vi "Test Multitone.vi"() -> ()   [LabVIEW 2019, in "Instrument.DAQ.lvclass"]
uses:
  Instrument.DAQ.lvclass
  <vilib>/measure/NI_MAPro.lvlib
  <vilib>/measure/NI_MABase.lvlib
panel:
  out "timer 0 (ms)":u32
  out "timer 3 (ms)":u32
  out "timer 2 (ms)":u32
  out "timer 1 (ms)":u32
  out "Waveform Graph":waveform(dbl)[](graph)
  out "resulting string":string
  in  "phase":dbl[](array[numeric])
  in  "frequency":dbl[](array[numeric])
  in  "amplitude":dbl[](array[numeric])
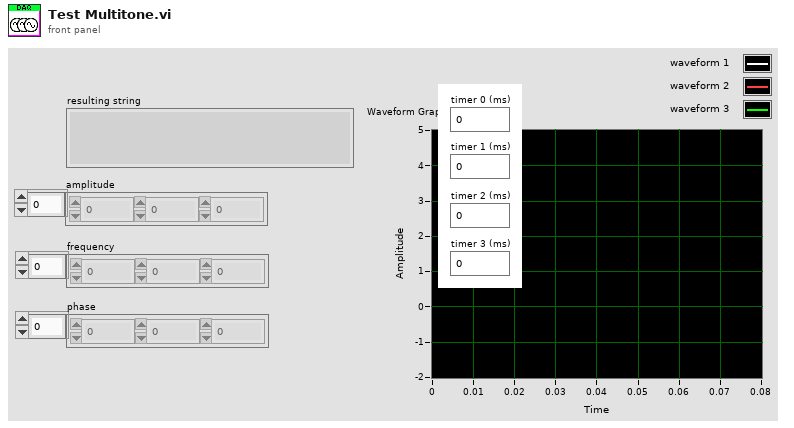
[diagram p1: front panel]
types:
  T1 = enum16{"Sine Wave", "Triangle Wave", "Square Wave", "Sawtooth Wave"}
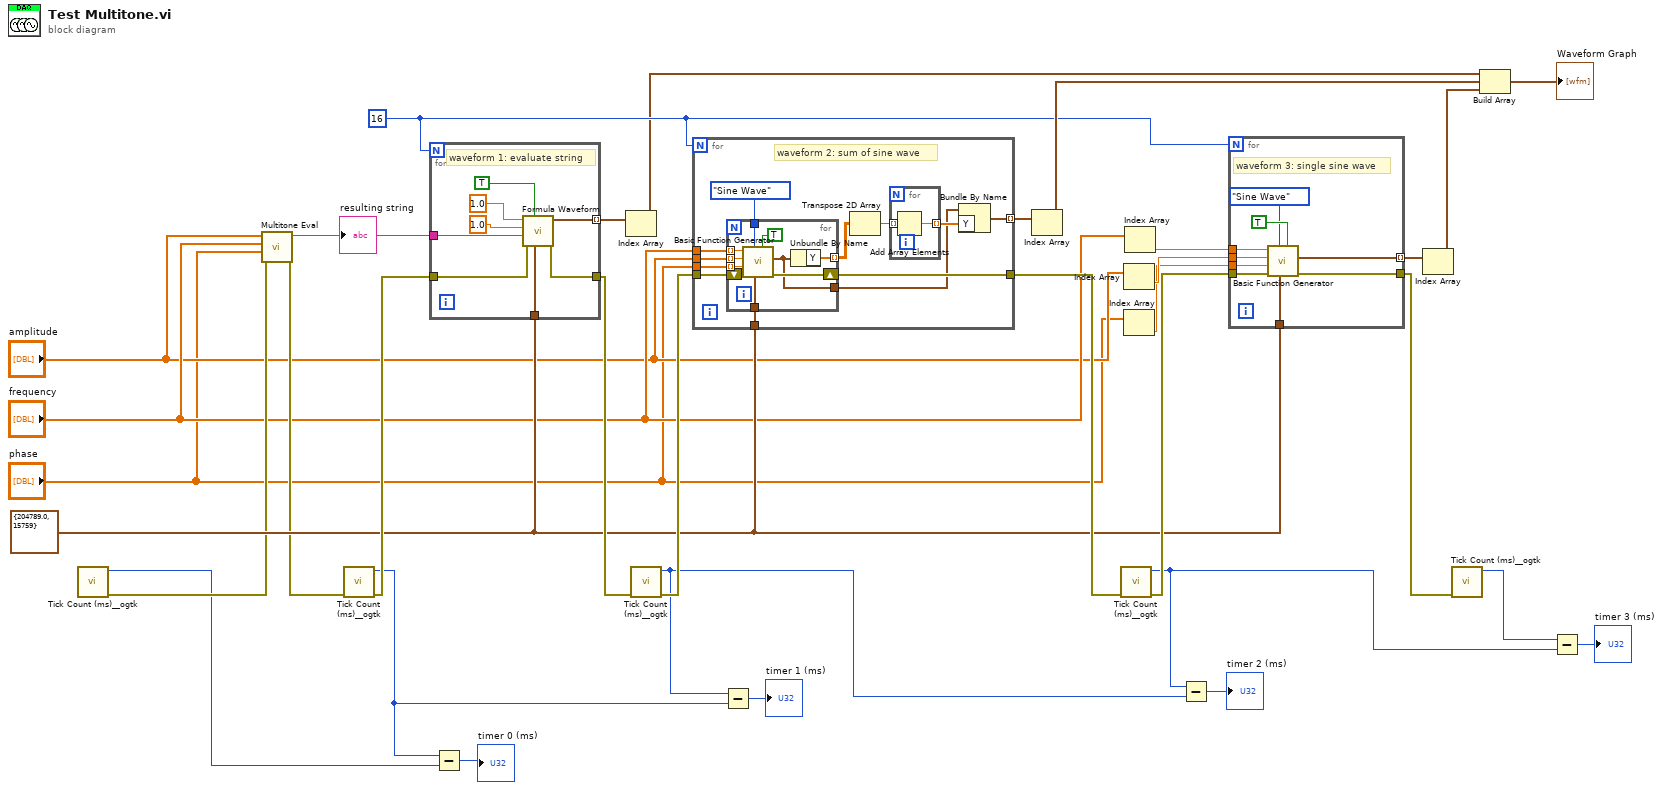
[diagram p0: block diagram]
diagram:
  w9 = 16
  w28 = cluster{"Fs":dbl, "#s":i32} {"Fs"=204789.0, "#s"=15759} ("sampling")
  n1 = call <userlib>:"Tick Count (ms)__ogtk.vi"() -> ("error out"=w26:errorcluster, "millisecond timer value"=w2:u32)  [unwired: 10 in]
  n2 = call "Multitone Eval.vi"("error in (no error)"=w26, "phase"="phase", "frequency"="frequency", "amplitude"="amplitude") -> ("error out"=w25:errorcluster, "String"=w24:string)  [unwired: 6 in]
  "resulting string" <- w24
  n3 = call <userlib>:"Tick Count (ms)__ogtk.vi"("error in (no error)"=w25) -> ("error out"=w33:errorcluster, "millisecond timer value"=w3:u32)  [unwired: 9 in]
  n4 = for {
    N: w9 -> [_]
    tunnel: w28 -> [w41]
    tunnel: w24 -> [w40]
    tunnel: w33 -> [w36]
    tunnel: [w35] -> w32
    tunnel: [w34] -> w23 mode=indexing
    # "waveform 1: evaluate string"
    n5 = call <vilib>:"Formula Waveform.vi"("sampling info"=w41, "reset signal"=TRUE, "error in (no error)"=w36, "formula"=w40, "amplitude"=1.0, "frequency"=1.0) -> ("error out"=w35:errorcluster, "signal out"=w34:waveform(dbl))  [unwired: 4 in]
  }
  n6 = Subtract(x=w3, y=w2) -> (x-y=→"timer 0 (ms)":u32)
  n7 = Index Array(array=w23) -> (element=w5:waveform(dbl))  [unwired: 1 in]
  n8 = call <userlib>:"Tick Count (ms)__ogtk.vi"("error in (no error)"=w32) -> ("error out"=w31:errorcluster, "millisecond timer value"=w6:u32)  [unwired: 9 in]
  n9 = for {
    N: w9 -> [_]
    tunnel: w31 -> [w53]
    tunnel: w28 -> [w52]
    tunnel: [w51] -> w30
    tunnel: "frequency" -> [w50]
    tunnel: "amplitude" -> [w49]
    tunnel: "phase" -> [w48]
    tunnel: [w45] -> w18 mode=indexing
    # "waveform 2: sum of sine wave"
    n10 = for {
      tunnel: w52 -> [w64]
      shift-right: [w63] -> w51
      shift-left: w53 -> [w65]
      tunnel: w50 -> [w62] mode=indexing
      tunnel: w49 -> [w61] mode=indexing
      tunnel: w48 -> [w60] mode=indexing
      tunnel: T1."Sine Wave" ("signal type") -> [w59]
      tunnel: [w58] -> w42 mode=indexing
      tunnel: [w57] -> w43
      n11 = call <vilib>:"Basic Function Generator.vi"("reset signal"=TRUE, "sampling info"=w64, "signal type"=w59, "error in (no error)"=w65, "phase"=w60, "amplitude"=w61, "frequency"=w62) -> ("error out"=w63:errorcluster, "signal out"=w57:waveform(dbl))  [unwired: 2 in, 1 out]
      n12 = Unbundle By Name(w57) -> ("Y"=w58:dbl[])
    }
    n13 = Transpose 2D Array(2D array=w42) -> (transposed array=w46:dbl[][])
    n14 = for {
      tunnel: w46 -> [w55] mode=indexing
      tunnel: [w54] -> w44 mode=indexing
      n15 = Add Array Elements(numeric array=w55) -> (sum=w54:dbl)
    }
    n16 = Bundle By Name(cluster=w43, "Y"=w44) -> (w45:waveform(dbl))
  }
  n17 = Subtract(x=w6, y=w3) -> (x-y=→"timer 1 (ms)":u32)
  n18 = Index Array(array=w18) -> (element=w11:waveform(dbl))  [unwired: 1 in]
  n19 = call <userlib>:"Tick Count (ms)__ogtk.vi"("error in (no error)"=w30) -> ("error out"=w29:errorcluster, "millisecond timer value"=w15:u32)  [unwired: 9 in]
  n20 = Index Array(array="amplitude") -> (element=w8:dbl)  [unwired: 1 in]
  n21 = Index Array(array="phase") -> (element=w7:dbl)  [unwired: 1 in]
  n22 = Index Array(array="frequency") -> (element=w21:dbl)  [unwired: 1 in]
  n23 = Subtract(x=w15, y=w6) -> (x-y=→"timer 2 (ms)":u32)
  n24 = for {
    N: w9 -> [_]
    tunnel: w29 -> [w74]
    tunnel: w28 -> [w73]
    tunnel: [w72] -> w27
    tunnel: w21 -> [w71]
    tunnel: [w68] -> w17 mode=indexing
    tunnel: w8 -> [w67]
    tunnel: w7 -> [w66]
    # "waveform 3: single sine wave"
    n25 = call <vilib>:"Basic Function Generator.vi"("reset signal"=TRUE, "sampling info"=w73, "signal type"=T1."Sine Wave", "error in (no error)"=w74, "phase"=w66, "amplitude"=w67, "frequency"=w71) -> ("error out"=w72:errorcluster, "signal out"=w68:waveform(dbl))  [unwired: 2 in, 1 out]
  }
  n26 = Index Array(array=w17) -> (element=w4:waveform(dbl))  [unwired: 1 in]
  n27 = call <userlib>:"Tick Count (ms)__ogtk.vi"("error in (no error)"=w27) -> ("millisecond timer value"=w16:u32)  [unwired: 9 in, 1 out]
  n28 = Build Array(w5, w11, w4) -> (→"Waveform Graph":waveform(dbl)[])
  n29 = Subtract(x=w16, y=w15) -> (x-y=→"timer 3 (ms)":u32)
